vi "数据查询_仪器数据.vi"() -> ()   [LabVIEW 2016]
uses:
  <vilib>/Utility/miscctls.llb/LVRowAndColumnUnsignedTypeDef.ctl
  <vilib>/Utility/miscctls.llb/LVPointTypeDef.ctl
  <userlib>/_OpenG.lib/array/array.llb/Sort 2D Array (String)__ogtk.vi
  <userlib>/_OpenG.lib/array/array.llb/Sort 1D Array (I32)__ogtk.vi
  <vilib>/regexp/Match Regular Expression.xnode
panel:
  out "condition":string
  out "显示项":string[](array[string])
  out "确定查询":bool
  in  "布尔":bool
  in  "条件筛选":bool
  in  "数据列表选择框":string(xcontrol)
  in  "导出":bool
  in  "数据表":T1
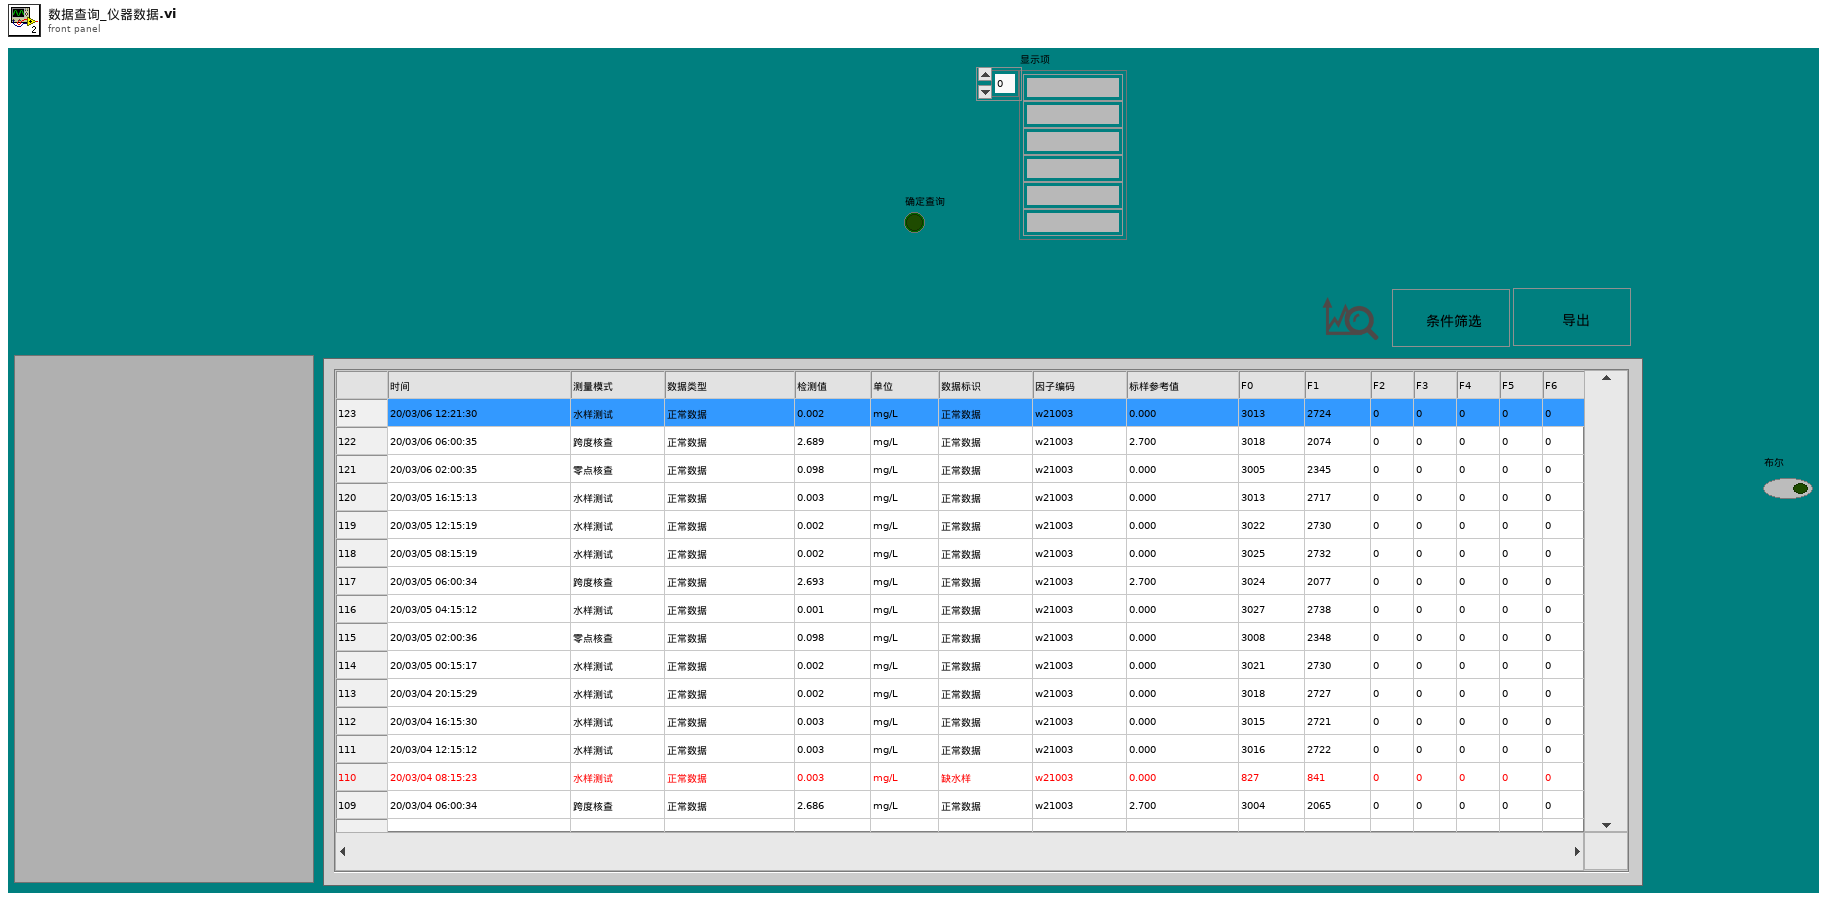
[diagram p1: front panel]
types:
  T1 = typedef "数据查询大列表框.ctl" = i32
  T2 = typedef "LVRowAndColumnUnsignedTypeDef.ctl" = cluster{"Row":u32, "Column":u32}
  T3 = typedef "LVPointTypeDef.ctl" = cluster{"Horizontal":i16, "Vertical":i16}
  T4 = enum8{"Enabled", "Disabled", "Disabled and Grayed Out"}
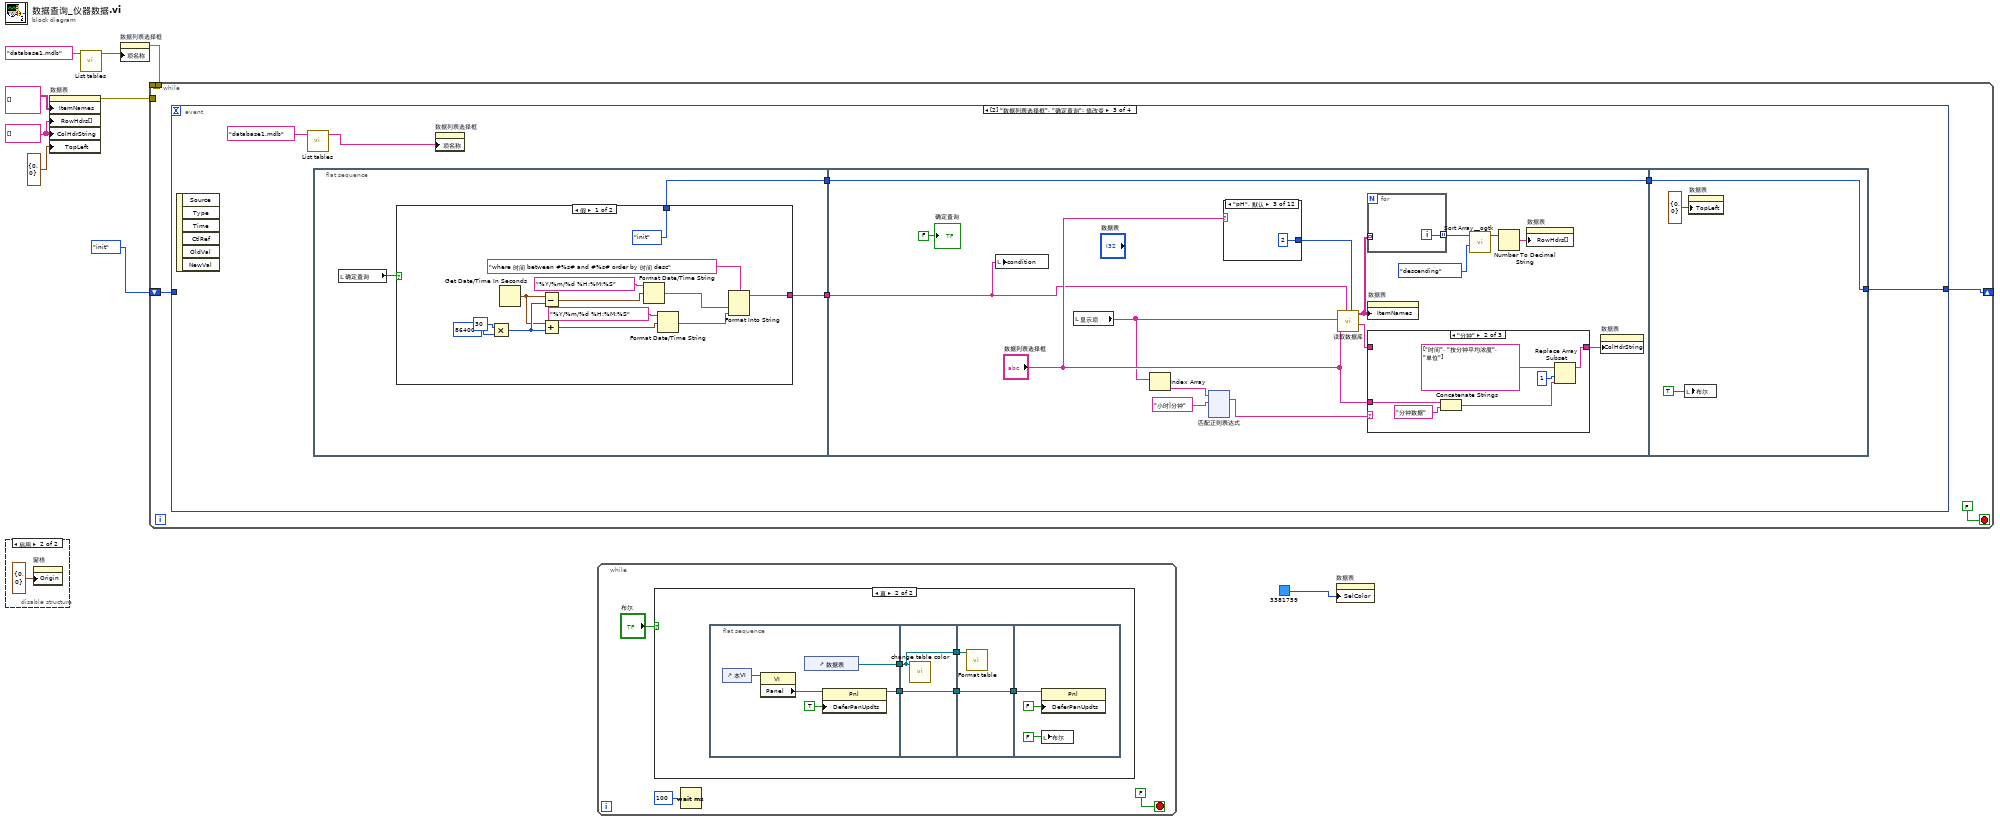
[diagram p0: block diagram]
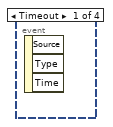
[diagram p3: hidden frame]
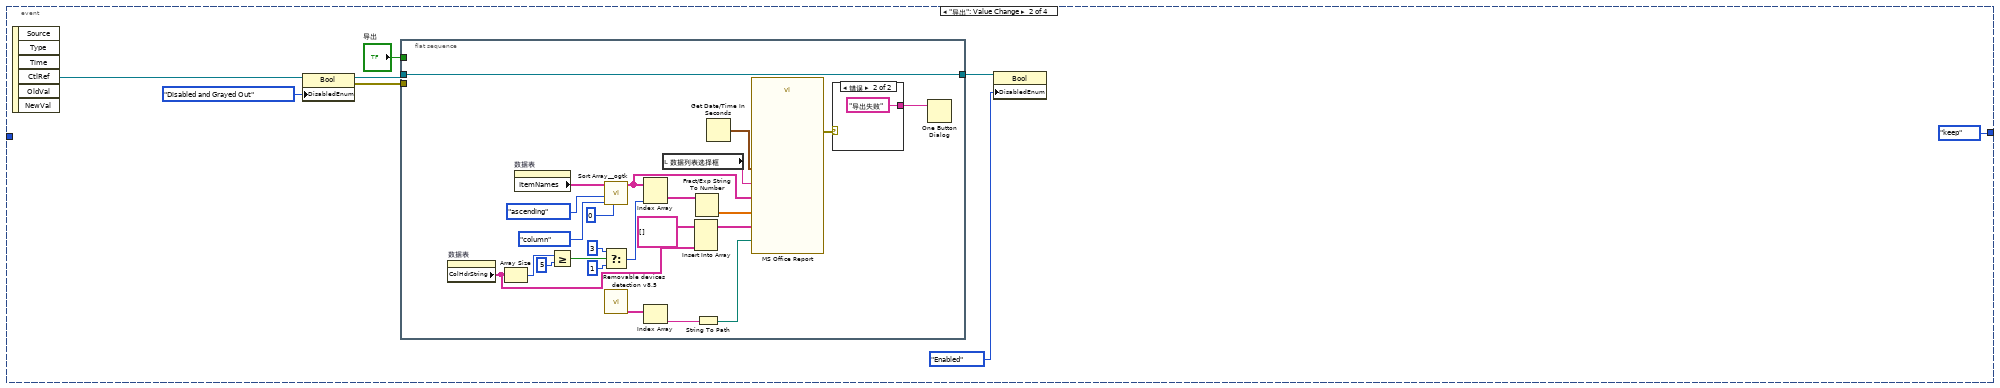
[diagram p4: hidden frame]
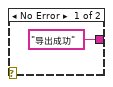
[diagram p5: hidden frame]
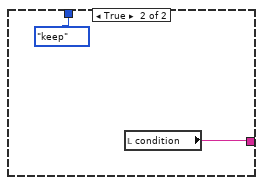
[diagram p6: hidden frame]
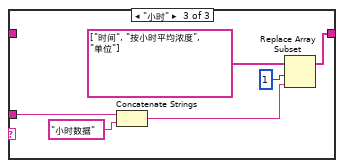
[diagram p8: hidden frame]
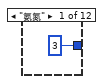
[diagram p9: hidden frame]
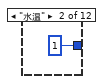
[diagram p10: hidden frame]
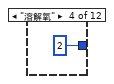
[diagram p11: hidden frame]
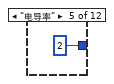
[diagram p12: hidden frame]
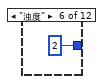
[diagram p13: hidden frame]
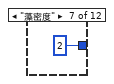
[diagram p14: hidden frame]
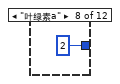
[diagram p15: hidden frame]
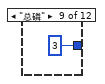
[diagram p16: hidden frame]
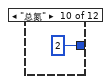
[diagram p17: hidden frame]
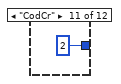
[diagram p18: hidden frame]
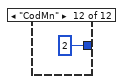
[diagram p19: hidden frame]
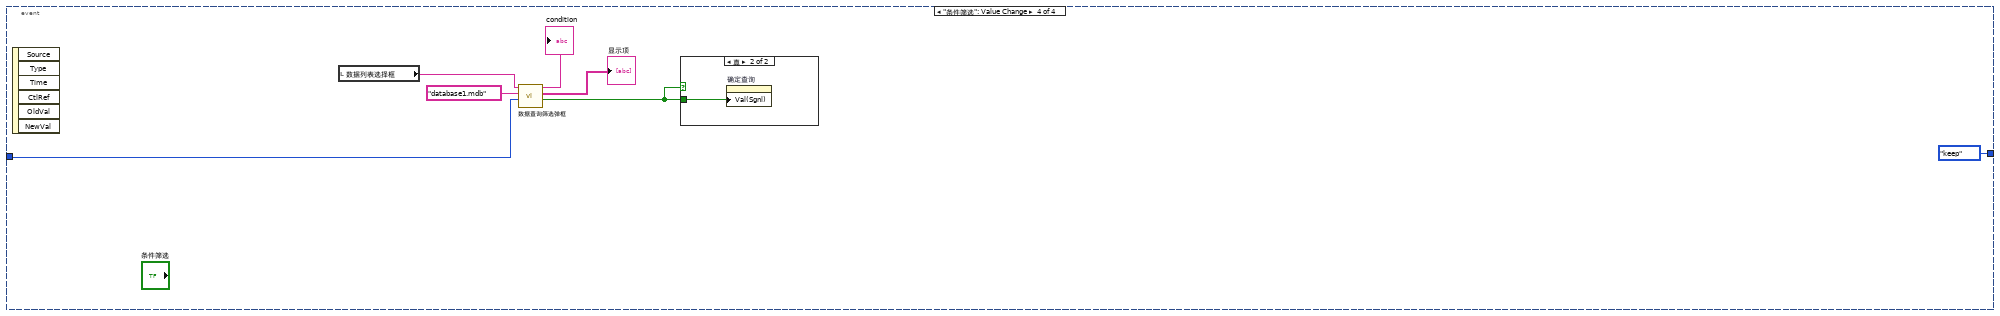
[diagram p20: hidden frame]
diagram:
  w6 = string[] [] ("行首字符串[]")
  n1 = disable-structure shown="启用" {
    frame Disabled {
    }
    frame Enabled {
      n2 = property on="窗格" class="Pane"("Origin"=T3 {"Horizontal"=0, "Vertical"=0} ("原点")) -> ()  [unwired: 2 in, 2 out]
    }
  }
  n3 = property on="数据表" class="MCListbox (严格)"("ItemNames"=string[][] [] ("项名"), "RowHdrs[]"=w6, "ColHdrString"=w6, "TopLeft"=T2 {"Row"=0, "Column"=0} ("左上可见单元格")) -> (error out=w8:errorcluster)  [unwired: 2 in, 1 out]
  n4 = call "List tables.vi"("database"="database1.mdb") -> ("tables"=w4:string[])  [unwired: 9 in, 1 out]
  n5 = property on="数据列表选择框" class="数据列表选择框 (严格)"("项名称"=w4) -> (error out=w2:errorcluster)  [unwired: 2 in, 1 out]
  n6 = while {
    tunnel: w8 -> [_]
    tunnel: [w13] -> _
    tunnel: w2 -> [w13]
    shift-right: [w11] -> _
    shift-left: enum16{"init", "keep"}."init" ("是否初始化") -> [w12]
    stop <- FALSE stop-if-true
    n7 = event shown="[2] \"数据列表选择框\", \"确定查询\": 值改变" {
      selector: _ -> [_ _ _ _]
      dyn-events: _ -> [_ _ _ _]
      timeout: _ -> [_ _ _ _]
      tunnel: w12 -> [_ _ _ w233]
      tunnel: [_ enum16{"init", "keep"}."keep" ("是否初始化") w51 enum16{"init", "keep"}."keep" ("是否初始化")] -> w11
      event Timeout {
        n8 = event-data() -> ()  [unwired: 1 in, 3 out]
      }
      event "导出": Value Change {
        n9 = event-data() -> ("CtlRef"=w16:refnum<vi>)  [unwired: 1 in, 5 out]
        n10 = property class="Bool"(reference=w16, "DisabledEnum"=T4."Disabled and Grayed Out" ("禁用")) -> (reference out=w20:refnum<vi>, error out=w21:errorcluster)  [unwired: 1 in]
        n11 = flat-sequence {
          tunnel: w21 -> [_]
          tunnel: [w38] -> w19
          tunnel: w20 -> [w38]
          tunnel: "导出" -> [_]
          frame #0 {
            n12 = property on="数据表" class="MCListbox (严格)"() -> ("ColHdrString"=w25:string[])  [unwired: 2 in, 2 out]
            n13 = Array Size(array=w25) -> (size(s)=w32:i32)
            n14 = property on="数据表" class="MCListbox (严格)"() -> ("ItemNames"=w23:string[][])  [unwired: 2 in, 2 out]
            n15 = Greater Or Equal?(x=w32, y=5) -> (x >= y?=w30:bool)
            n16 = call-poly <userlib>:"Sort Array__ogtk.vi"("Column/Row to Sort By"=u32 0, "Sort By in"=enum16{"row", "column"}."column", "Order"=enum16{"ascending", "descending"}."ascending", "Array in"=w23) -> ("Sorted Array out"=w45:string[][])  [unwired: 4 in, 3 out]
            n17 = Select(t=3 ("禁用的索引 (列)"), s=w30, f=1) -> (s? t:f=w28:i32)
            n18 = call "Removable devices detection v8.5.vi"() -> ("Removable"=w35:string[])  [unwired: 4 out]
            n19 = Index Array(array=w45, index (col)=w28) -> (element=w41:string[])  [unwired: 1 in]
            n20 = Index Array(array=w35) -> (element=w34:string)  [unwired: 1 in]
            n21 = local read "数据列表选择框"() -> (w39:string)
            n22 = Insert Into Array(array=string[][] [], new element=w25) -> (w24:string[][])  [unwired: 2 in]
            n23 = Fract/Exp String To Number(string=w41) -> (number=w40:dbl[])  [unwired: 3 in, 1 out]
            n24 = String To Path(string=w34) -> (path=w33:path)
            n25 = Get Date/Time In Seconds() -> (seconds since 1Jan1904=w46:timestamp)
            n26 = call "MS Office Report"("Path to Save Report"=w33, "导出日期"=w46, "监测参数"=w39, "数据输入"=w45, "图表输入"=w40, "字段定义"=w24) -> ("error out"=w37:errorcluster)  [unwired: 20 in, 1 out]
            n27 = case shown="错误" w37 {
              tunnel: ["导出成功" ("消息") "导出失败" ("消息")] -> w36
              frame No Error {
              }
              frame Error {
              }
            }
            n28 = One Button Dialog(message=w36) -> ()  [unwired: 1 in, 1 out]
          }
        }
        n29 = property class="Bool"(reference=w19, "DisabledEnum"=T4."Enabled" ("禁用")) -> ()  [unwired: 1 in, 2 out]
      }
      event "数据列表选择框", "确定查询": Value Change {
        n30 = event-data() -> ()  [unwired: 1 in, 6 out]
        n31 = call "List tables.vi"("database"="database1.mdb") -> ("tables"=w53:string[])  [unwired: 9 in, 1 out]
        n32 = flat-sequence {
          tunnel: [w56] -> w52
          tunnel: [w55] -> w49
          tunnel: w52 -> [w74]
          tunnel: [w73] -> w50
          tunnel: w49 -> [w73]
          tunnel: [w229] -> w51
          tunnel: w50 -> [w229]
          frame #0 {
            n33 = local read "确定查询"() -> (w57:bool)
            n34 = case shown="假" w57 {
              tunnel: [w59 w72] -> w56
              tunnel: [enum16{"init", "keep"}."init" ("是否初始化") enum16{"init", "keep"}."keep" ("是否初始化")] -> w55
              frame False {
                n35 = Multiply(x=30, y=86400) -> (x*y=w61:i32)
                n36 = Get Date/Time In Seconds() -> (seconds since 1Jan1904=w60:timestamp)
                n37 = Subtract(x=w60, y=w61) -> (x-y=w67:timestamp)
                n38 = Add(x=w60, y=w61) -> (x+y=w66:timestamp)
                n39 = Format Date/Time String(time format string (%c)="%Y/%m/%d %H:%M:%S" ("时间格式字符串(%c)"), seconds (now)=w67) -> (date/time string=w69:string)  [unwired: 1 in]
                n40 = Format Date/Time String(time format string (%c)="%Y/%m/%d %H:%M:%S" ("时间格式字符串(%c)"), seconds (now)=w66) -> (date/time string=w70:string)  [unwired: 1 in]
                n41 = Format Into String(format string="where 时间 between #%s# and #%s# order by 时间 desc", w69, w70) -> (resulting string=w59:string)  [unwired: 2 in, 1 out]
              }
              frame True {
                n42 = local read "condition"() -> (w72:string)
              }
            }
          }
          frame #1 {
            n43 = local write "condition"(w74) -> ()
            n44 = local read "显示项"() -> (w79:string[])
            n45 = Index Array(array=w79) -> (element=w77:string)  [unwired: 1 in]
            n46 = xnode "匹配正则表达式"("输入字符串"=w77, "正则表达式"="小时|分钟") -> ("所有匹配"=w76:string)  [unwired: 4 in, 4 out]
            n47 = case shown="\"pH\", 默认" "数据列表选择框" {
              tunnel: [i16 3 ("精度(6)") i16 1 ("精度(6)") i16 2 ("精度(6)") i16 2 ("精度(6)") i16 2 ("精度(6)") i16 2 ("精度(6)") i16 2 ("精度(6)") i16 2 ("精度(6)") i16 3 ("精度(6)") i16 2 ("精度(6)") i16 2 ("精度(6)") i16 2 ("精度(6)")] -> w86
              frame "氨氮" {
              }
              frame "水温" {
              }
              frame "pH", Default {
              }
              frame "溶解氧" {
              }
              frame "电导率" {
              }
              frame "浊度" {
              }
              frame "藻密度" {
              }
              frame "叶绿素a" {
              }
              frame "总磷" {
              }
              frame "总氮" {
              }
              frame "CodCr" {
              }
              frame "CodMn" {
              }
            }
            n48 = call "读取数据库.vi"("精度(6)"=w86, "condition"=w74, "显示项"=w79, "组合框"="数据列表选择框") -> ("columns"=w85:string[], "表格"=w81:string[][])  [unwired: 4 in, 2 out]
            n49 = for {
              tunnel: w81 -> [_] mode=indexing
              tunnel: [w228] -> w88 mode=indexing
              i -> [w228]
            }
            n50 = property on="数据表" class="MCListbox (严格)"("ItemNames"=w81) -> ()  [unwired: 2 in, 2 out]
            n51 = case shown="\"分钟\"" w76 {
              tunnel: w85 -> [w203 _ _]
              tunnel: [w203 w207 w211] -> w84
              tunnel: "数据列表选择框" -> [_ w206 w212]
              frame Default {
              }
              frame "分钟" {
                n52 = Concatenate Strings(w206, "分钟数据" ("字符串")) -> (w204:string)
                n53 = Replace Array Subset(array=string[] ["时间", "按分钟平均浓度", "单位"] ("columns"), new element=w204, index=1 ("索引")) -> (w207:string[])
              }
              frame "小时" {
                n54 = Concatenate Strings(w212, "小时数据" ("字符串")) -> (w213:string)
                n55 = Replace Array Subset(array=string[] ["时间", "按小时平均浓度", "单位"] ("columns"), new element=w213, index=1 ("索引")) -> (w211:string[])
              }
            }
            n56 = call-poly <userlib>:"Sort Array__ogtk.vi"("Order"=enum16{"ascending", "descending"}."descending", "Array in"=w88) -> ("Sorted Array out"=w82:i32[])  [unwired: 8 in, 1 out]
            n57 = Number To Decimal String(number=w82) -> (decimal integer string=w87:string[])  [unwired: 1 in]
            n58 = property on="数据表" class="MCListbox (严格)"("RowHdrs[]"=w87) -> ()  [unwired: 2 in, 2 out]
            n59 = property on="数据表" class="MCListbox (严格)"("ColHdrString"=w84) -> ()  [unwired: 2 in, 2 out]
            "确定查询" <- FALSE ("确定查询")
          }
          frame #2 {
            n60 = local write "布尔"(TRUE ("布尔")) -> ()
            n61 = property on="数据表" class="MCListbox (严格)"("TopLeft"=T2 {"Row"=0, "Column"=0} ("索引值")) -> ()  [unwired: 2 in, 2 out]
          }
        }
        n62 = property on="数据列表选择框" class="数据列表选择框 (严格)"("项名称"=w53) -> ()  [unwired: 2 in, 2 out]
      }
      event "条件筛选": Value Change {
        n63 = event-data() -> ()  [unwired: 1 in, 6 out]
        n64 = local read "数据列表选择框"() -> (w237:string)
        n65 = call "数据查询筛选弹框.vi"("是否初始化"=w233, "database"="database1.mdb", "table"=w237) -> ("确定输出"=w234:bool, "显示项"=→"显示项":string[], "condition"=→"condition":string)  [unwired: 5 in, 1 out]
        n66 = case shown="真" w234 {
          tunnel: w234 -> [_ w239]
          frame False {
          }
          frame True {
            n67 = property on="确定查询" class="Bool (严格)"("Val(Sgnl)"=w239) -> ()  [unwired: 2 in, 2 out]
          }
        }
      }
    }
  }
  n68 = while {
    stop <- FALSE stop-if-true
    n69 = case shown="真" "布尔" {
      frame False {
      }
      frame True {
        n70 = flat-sequence {
          tunnel: [w249] -> w245
          tunnel: [w248] -> w244
          tunnel: [w254] -> w246
          tunnel: w245 -> [w254]
          tunnel: w244 -> [w253]
          tunnel: [w253] -> w243
          tunnel: [w256] -> w247
          tunnel: w246 -> [w256]
          tunnel: w243 -> [w255]
          tunnel: w247 -> [w259]
          frame #0 {
            n71 = control-ref of="本VI"() -> (w250:refnum<vi>)
            n72 = property class="VI"(reference=w250) -> ("Panel"=w251:refnum<vi>)  [unwired: 1 in, 2 out]
            n73 = control-ref of="数据表"() -> (w248:refnum<vi>)
            n74 = property class="Pnl"(reference=w251, "DeferPanUpdts"=TRUE ("延迟前面板更新")) -> (reference out=w249:refnum<vi>)  [unwired: 1 in, 1 out]
          }
          frame #1 {
            n75 = call "change table color.vi"("MulticolumnListbox输入"=w253) -> ()  [unwired: 11 in]
          }
          frame #2 {
            n76 = call "Format table.vi"("Table输入"=w255) -> ()  [unwired: 11 in]
          }
          frame #3 {
            n77 = property class="Pnl"(reference=w259, "DeferPanUpdts"=FALSE ("延迟前面板更新")) -> ()  [unwired: 1 in, 2 out]
            n78 = local write "布尔"(FALSE ("布尔")) -> ()
          }
        }
      }
    }
    n79 = Wait (ms)(milliseconds to wait=u32 100 ("等待时间（毫秒）")) -> ()  [unwired: 1 out]
  }
  n80 = property on="数据表" class="MCListbox (严格)"("SelColor"=u32 3381759) -> ()  [unwired: 2 in, 2 out]
